vi "Get Errno Value for Calling Thread.vi"(8 "error in":errorcluster) -> (0 "error out":errorcluster, 2 "errno number":i32, 3 "errno":T1(ring))   [LabVIEW 2018, in "PCANBasic.lvlib" / "epoll.lvclass"]
uses:
  epoll.lvclass
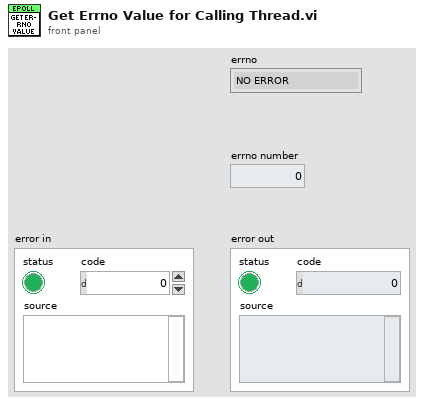
[diagram p1: front panel]
types:
  T1 = enum16{"NO ERROR", "EPERM", "ENOENT", "ESRCH", "EINTR", "EIO", "ENXIO", "E2BIG", "ENOEXEC", "EBADF", "ECHILD", "EAGAIN", "ENOMEM", "EACCES", "EFAULT", "ENOTBLK", "EBUSY", "EEXIST", "EXDEV", "ENODEV", "ENOTDIR", "EISDIR", "EINVAL", "ENFILE", "EMFILE", "ENOTTY", "ETXTBSY", "EFBIG", "ENOSPC", "ESPIPE", "EROFS", "EMLINK", "EPIPE", "EDOM", "ERANGE", "EDADLK", "ENAMETOOLONG", "ENOLCK", "ENOSYS", "ENOTEMPTY", "ELOOP", "EWOULDBLOCK", "ENOMSG", "EIDRM", "ECHRNG", "EL2NSYNC", "EL3HLT", "EL3RST", "ELNRNG", "EUNATCH", "ENOCSI", "EL2HLT", "EBADE", "EBADR", "EXFULL", "ENOANO", "EBADRQC", "EBADSLT", "EDEADLOCK", "EBFONT", "ENOSTR", "ENODATA", "ETIME", "ENOSR", "ENONET", "ENOPKG", "EREMOTE", "ENOLINK", "EADV", "ESRMNT", "ECOMM", "EPROTO", "EMULTIHOP", "EDOTDOT", "EBADMSG", "EOVERFLOW", "ENOTUNIQ", "EBADFD", "EREMCHG", "ELIBACC", "ELIBBAD", "ELIBSCN", "ELIBMAX", "ELIBEXEC", "ELISEQ", "ERESTART", "ESTRPIPE", "EUSERS", "ENOTSOCK", "EDESTADDRREQ", "EMSGSIZE", "EPROTOTYPE", "ENOPROTOOPT", "EPROTONOSUPPORT", "ESOCKTNOSUPPORT", "EOPNOTSUPP", "EPFNOSUPPORT", "EAFNOSUPPORT", "EADDRINUSE", "EADDRNOTAVAIL", "ENETDOWN", "ENETUNREACH", "ENETRESET", "ECONNABORTED", "ECONNRESET", "ENOBUFS", "EISCONN", "ENOTCONN", "ESHUTDOWN", "ETOOMANYREFS", "ETIMEDOUT", "ECONNREFUSED", "EHOSTDOWN", "EHOSTUNREACH", "EALREADY", "EINPROGRESS", "ESTALE", "EUCLEAN", "ENOTNAM", "ENAVAIL", "EISNAM", "EREMOTEIO", "EDQUOT", "ENOMEDIUM", "EMEDIUMTYPE", "ECANCELED", "ENOKEY", "EKEYEXPIRED", "EKEYREVOKED", "EKEYREJECTED", "EOWNERDEAD", "ENOTRECOVERABLE", "ERFKILL", "EHWPOISON", "UNDEFINED"}
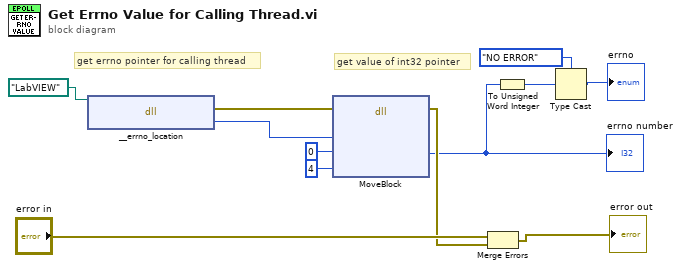
[diagram p0: block diagram]
diagram:
  # "get value of int32 pointer"
  # "get errno pointer for calling thread"
  n1 = dll-call lib="?" fn="__errno_location" ("get errno pointer for calling thread")(path in=path "LabVIEW") -> (error out=w11:errorcluster, "return type"=w12:u64)  [unwired: 2 in, 1 out]
  n2 = dll-call lib="LabVIEW" fn="MoveBlock"(error in=w11, "pointer"=w12, "data"=0, "size"=u64 4) -> (error out=w4:errorcluster, "data"=w2:i32)  [unwired: 5 in, 1 out]
  "errno number" <- w2
  n3 = Merge Errors("error in", w4) -> (→"error out":errorcluster)
  n4 = To Unsigned Word Integer(number=w2) -> (unsigned 16bit integer=w8:u16)
  n5 = Type Cast(type=T1."NO ERROR" ("errno"), x=w8) -> (*(type *) &x=→"errno":T1)
